vi "TCP Timeout - Amium.vi"(6 "Aktionen Timeout":T1, 9 "Timeout lesen":i32=110, 11 "Timeout schreiben":i32=190) -> (1 "Timeout lesen":i32=110, 3 "Timeout schreiben":i32=190)   [LabVIEW 2020, in "Amium PNS.lvlib" / "AK Kommunikation.lvlib"]
uses:
  AK Kommunikation.lvlib
  TCP Timeout Aktionen - Amium.ctl
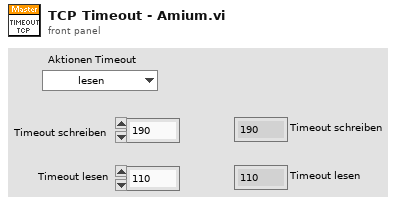
[diagram p1: front panel]
types:
  T1 = typedef "Amium PNS.lvlib/AK Kommunikation.lvlib/TCP Timeout Aktionen - Amium.ctl" = enum16{"lesen", "setzen"}
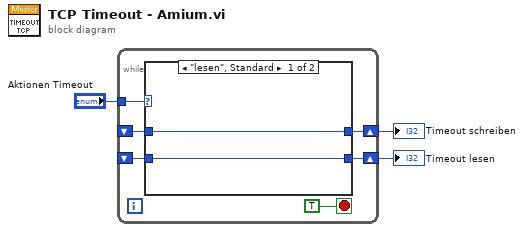
[diagram p0: block diagram]
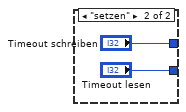
[diagram p2: hidden frame]
diagram:
  n1 = while {
    tunnel: "Aktionen Timeout" -> [w7]
    shift-right: [w9] -> w3
    shift-left: _ -> [w5]
    shift-right: [w8] -> w2
    shift-left: _ -> [w6]
    stop <- TRUE stop-if-true
    n2 = case shown="\"lesen\", Standard" w7 {
      tunnel: [w11 "Timeout schreiben"] -> w9
      tunnel: [w10 "Timeout lesen"] -> w8
      tunnel: w6 -> [w10 _]
      tunnel: w5 -> [w11 _]
      frame "lesen", Default {
      }
      frame "setzen" {
      }
    }
  }
  "Timeout schreiben" <- w3
  "Timeout lesen" <- w2
